vi "Platform data parsing.vi"(3 "Platform Data":string) -> (0 "Encoder":i64, 1 "Platform Data Array":i64[](array[numeric]))   [LabVIEW 2016]
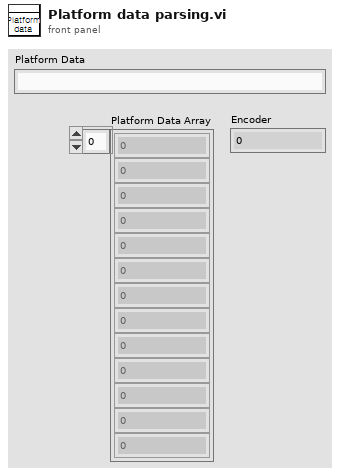
[diagram p1: front panel]
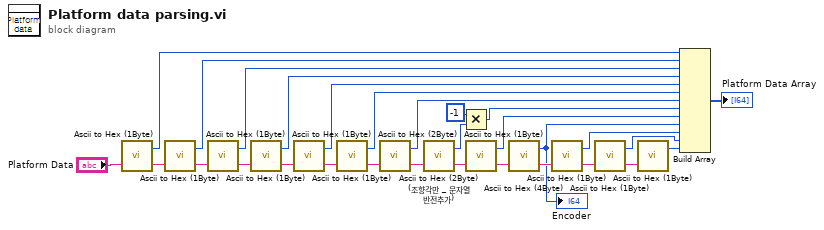
[diagram p0: block diagram]
diagram:
  n1 = call "Ascii to Hex (1Byte).vi"("Ascii 1"="Platform Data") -> ("Ascii 2"=w28:string, "Decimal"=w19:u32)  [unwired: 1 in]
  n2 = call "Ascii to Hex (1Byte).vi"("Ascii 1"=w28) -> ("Ascii 2"=w27:string, "Decimal"=w18:u32)  [unwired: 1 in]
  n3 = call "Ascii to Hex (1Byte).vi"("Ascii 1"=w27) -> ("Ascii 2"=w26:string, "Decimal"=w17:u32)  [unwired: 1 in]
  n4 = call "Ascii to Hex (1Byte).vi"("Ascii 1"=w26) -> ("Ascii 2"=w25:string, "Decimal"=w16:u32)  [unwired: 1 in]
  n5 = call "Ascii to Hex (1Byte).vi"("Ascii 1"=w25) -> ("Ascii 2"=w24:string, "Decimal"=w15:u32)  [unwired: 1 in]
  n6 = call "Ascii to Hex (1Byte).vi"("Ascii 1"=w24) -> ("Ascii 2"=w23:string, "Decimal"=w14:u32)  [unwired: 1 in]
  n7 = call "Ascii to Hex (2Byte).vi"("Ascii 1"=w23) -> ("Ascii 2"=w1:string, "Decimal"=w6:i16)  [unwired: 1 in]
  n8 = call "Ascii to Hex (2Byte) (조향각만 _ 문자열 반전추가).vi"("Ascii 1"=w1) -> ("Ascii 2"=w2:string, "Decimal"=w3:i16)  [unwired: 1 in]
  n9 = Multiply(x=i16 -1, y=w3) -> (x*y=w4:i16)
  n10 = call "Ascii to Hex (1Byte).vi"("Ascii 1"=w2) -> ("Ascii 2"=w22:string, "Decimal"=w13:u32)  [unwired: 1 in]
  n11 = call "Ascii to Hex (4Byte).vi"("Ascii 1"=w22) -> ("Ascii 2"=w20:string, "Decimal (4Byte)"=w7:i64)  [unwired: 1 in]
  "Encoder" <- w7
  n12 = call "Ascii to Hex (1Byte).vi"("Ascii 1"=w20) -> ("Ascii 2"=w21:string, "Decimal"=w12:u32)  [unwired: 1 in]
  n13 = call "Ascii to Hex (1Byte).vi"("Ascii 1"=w21) -> ("Ascii 2"=w9:string, "Decimal"=w11:u32)  [unwired: 1 in]
  n14 = call "Ascii to Hex (1Byte).vi"("Ascii 1"=w9) -> ("Decimal"=w8:u32)  [unwired: 1 in, 1 out]
  n15 = Build Array(w19, w18, w17, w16, w15, w14, w6, w4, w13, w7, w12, w11, w8) -> (→"Platform Data Array":i64[])
